vi "Host Write Configuration.vi"(3 "Host IP Address":string="10.0.22.186") -> ()   [LabVIEW 2013]
uses:
  <vilib>/Utility/config.llb/Write Key (String).vi
  <vilib>/Utility/config.llb/NI_LVConfig.lvlib
panel:
  in  "configuration file path":path=path "c:/clientconfig.ini"
  # "Set host IP address"
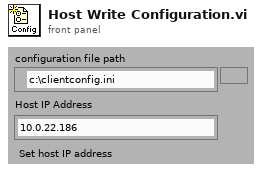
[diagram p1: front panel]
types:
  T1 = typedef "NI_LVConfig.lvlib/Config Data RefNum.ctl" = refnum<k1>
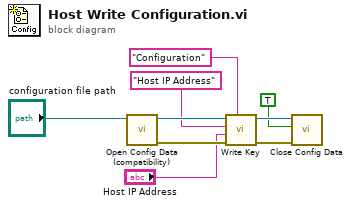
[diagram p0: block diagram]
diagram:
  n1 = call <vilib>:"Open Config Data (compatibility).vi"("configuration file path"="configuration file path") -> ("error out"=w8:errorcluster, "refnum"=w7:T1)  [unwired: 8 in, 1 out]
  n2 = call-poly <vilib>:"Write Key.vi"("section"="Configuration", "error in (no error)"=w8, "value"="Host IP Address", "key"="Host IP Address", "refnum"=w7) -> ("error out"=w6:errorcluster, "refnum out"=w5:T1)  [unwired: 1 in, 4 out]
  n3 = call <vilib>:"Close Config Data.vi"("error in (no error)"=w6, "write file if changed (T)"=TRUE ("write configuration file? (T)"), "refnum"=w5) -> ()  [unwired: 9 out]
